vi "Get User Input.vi"(9 "Location":u16(ring) items=["Austin, TX", "New York City, NY", "Chicago, IL"], 10 "Gender":enum32{"Radio Selection 1", "Radio Selection 2"}(radio), 11 "Name":string) -> (1 "Location":u16(ring) items=["Austin, TX", "New York City, NY", "Chicago, IL"], 2 "Gender":enum32{"Radio Selection 1", "Radio Selection 2"}(ring), 3 "Name":string)   [LabVIEW 2024]
panel:
  in  "Cancel":bool
  in  "OK":bool
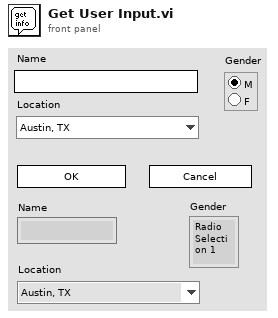
[diagram p1: front panel]
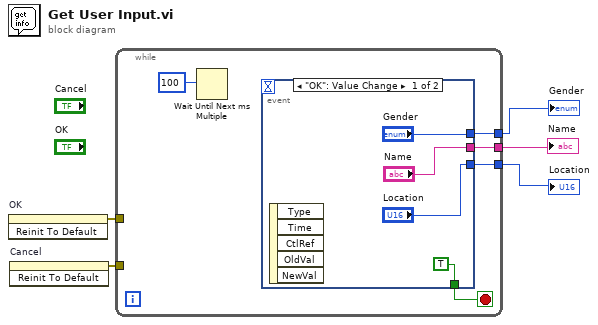
[diagram p0: block diagram]
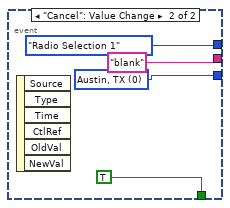
[diagram p2: hidden frame]
diagram:
  n1 = invoke on="OK" class="Bool" method="Reinit To Default"() -> (error out=w4:errorcluster)  [unwired: 3 in, 2 out]
  n2 = invoke on="Cancel" class="Bool" method="Reinit To Default"() -> (error out=w3:errorcluster)  [unwired: 3 in, 2 out]
  n3 = while {
    tunnel: [w10] -> w2
    tunnel: [w9] -> w5
    tunnel: [w8] -> w1
    tunnel: w4 -> [_]
    tunnel: w3 -> [_]
    stop <- w6 stop-if-true
    n4 = Wait Until Next ms Multiple(millisecond multiple=100) -> ()  [unwired: 1 out]
    n5 = event shown="[0] \"OK\": Value Change" {
      selector: _ -> [_ _]
      dyn-events: _ -> [_ _]
      timeout: _ -> [_ _]
      tunnel: [TRUE TRUE] -> w6
      tunnel: ["Gender" enum32{"Radio Selection 1", "Radio Selection 2"}."Radio Selection 1" ("Gender")] -> w10
      tunnel: ["Name" "blank" ("Name")] -> w9
      tunnel: ["Location" w15] -> w8
      event "OK": Value Change {
        n6 = event-data() -> ()  [unwired: 6 out]
      }
      event "Cancel": Value Change {
        w15 = u16 0 items=["Austin, TX", "New York City, NY", "Chicago, IL"] ("Location")
        n7 = event-data() -> ()  [unwired: 7 out]
      }
    }
  }
  "Name" <- w5
  "Gender" <- w2
  "Location" <- w1
